vi "Na-DAS_7609.vi"() -> (0 "DAQ Error":errorcluster)   [LabVIEW 2015]
doc: "Use this plug-in with the Nathan 7609 data acquisition system"
uses:
  Globals/Meas_global.vi
  PWA/PWAtasksGLOBAL.vi
  Globals/Extra_Commands_Global.vi
  Globals/Dynamic_call_global.ph.vi
  Globals/Trav_pos_global.vi
panel:
  in  "Input voltage range (V)":u8(ring)=1 items=["-5... +5 V", "-10... +10 V"]
  out "Config read-back ok":bool
  out "Overruns":u32
  # "PN 25/11/2014, 19/12/2014, 15/02/2015 (channels in any order), 17/08/2015 (stop ack mod)"
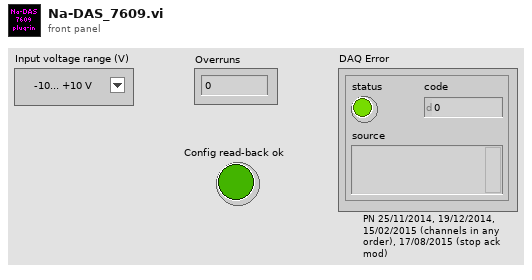
[diagram p1: front panel]
types:
  T1 = typedef "LDA_Setup.ctl" = cluster{"dimensions":enum16{"1D", "2D"}, "Analogue Freq Multiplier":dbl}
  T2 = typedef "Ch_and_Spans.ctl" = cluster{"high limit (10V)":sgl, "low limit (-10V)":sgl, "Ch No":i16, "Var name":string, "Use Latest Calib":bool}
  T3 = typedef "Traverse_cluster.ctl" = cluster{"Start X":sgl, "Start Y":sgl, "Start Z":sgl, "End X":sgl, "End Y":sgl, "End Z":sgl, "No. of pts.":i32, "Spacing":T4, "Filename":path, "Tunnel Speed":dbl, "Averaging time (min)":dbl, "Extra Commands":string, "Carrier_1 Q (l/min)":dbl, "Carrier_2 Q (l/min)":dbl, "Trace Gas Concentration (%)":dbl, "Specific Arguments":string, "Comments":string, "Row No":i32, "Row Type Selector":T5, "Completion time":string, "Row Duration (mins)":dbl, "No. of Valid pts.":i32, "Meas Setup File":string}
  T4 = typedef "Spacing.ctl" = enum16{"Linear", "Log", "Gauss", "Specified", "N/A"}
  T5 = typedef "Multi_run_mode.ctl" = enum16{"Move Traverse Only", "Set Tunnel Speed Only", "Set Source Only", "Set Measurement Conditions", "Single Measurement", "Vertical Profile", "Lateral Profile", "Longitudinal Profile", "Explore Volume", "Multi-Axis Profile", "Auto Calibrate", "Meas Fast FID Bkgnd", "Check Beam Power", "Scanning Valve Measurement", "Run VI Named:", "Set ADAM Ch", "Wait (minutes)", "Send Message", "Synchronize With:", "Fall Back to this Row", "Turn Off Row Repeating", "Blank Row", "Traverse 3D Volume"}
  T6 = typedef "Trigger_Mode.ctl" = enum16{"Free Running", "Start on Trigger", "Trigger Every Block", "Trigger Every Sample"}
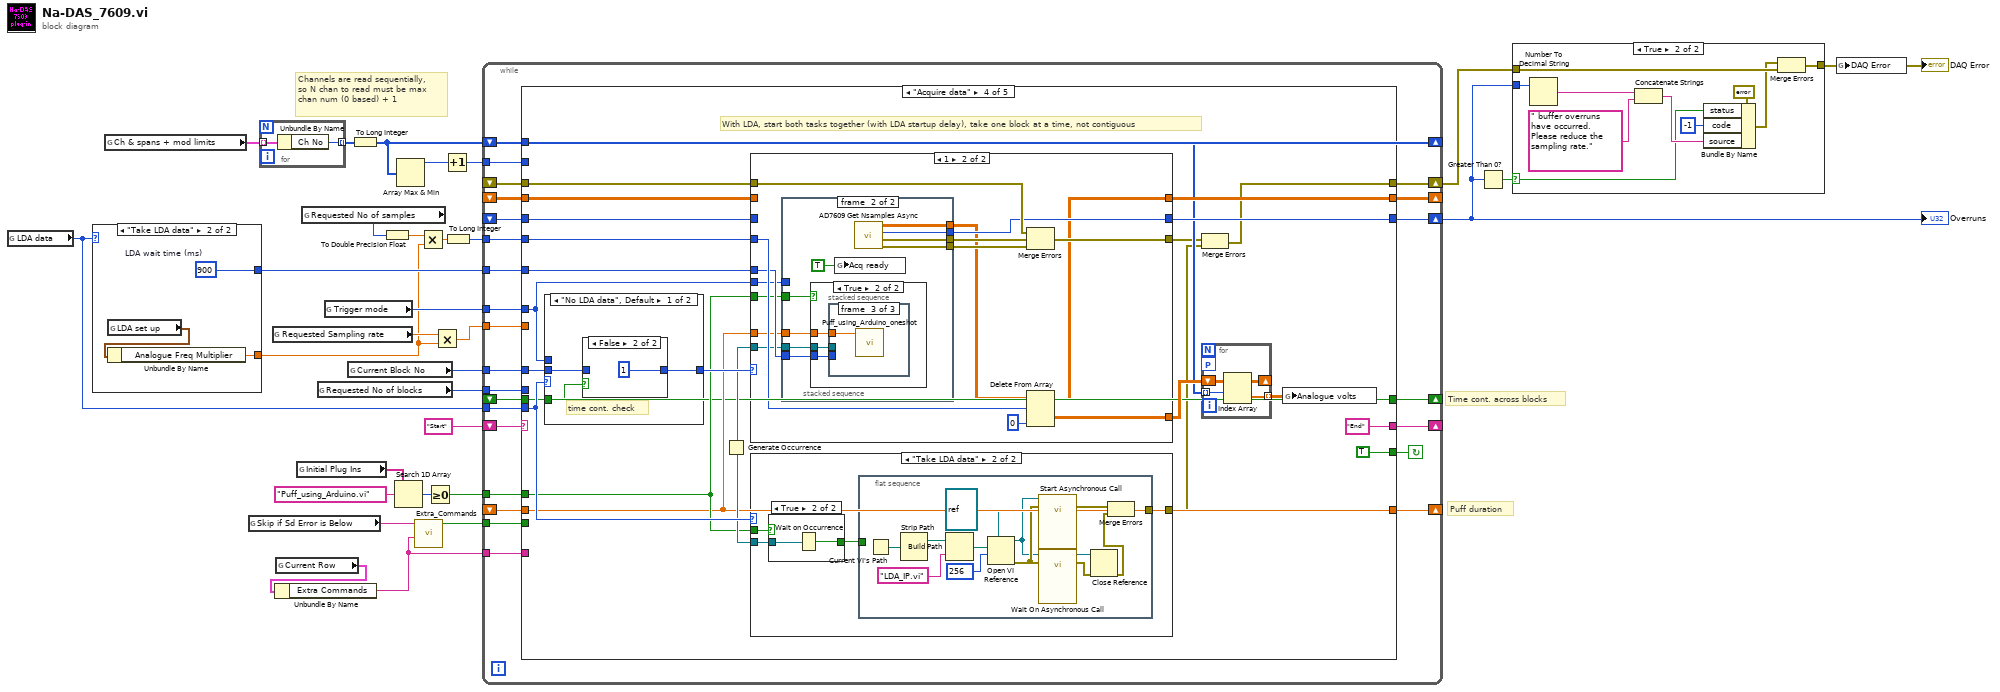
[diagram p0: block diagram]
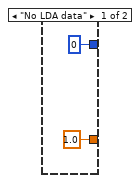
[diagram p3: hidden frame]
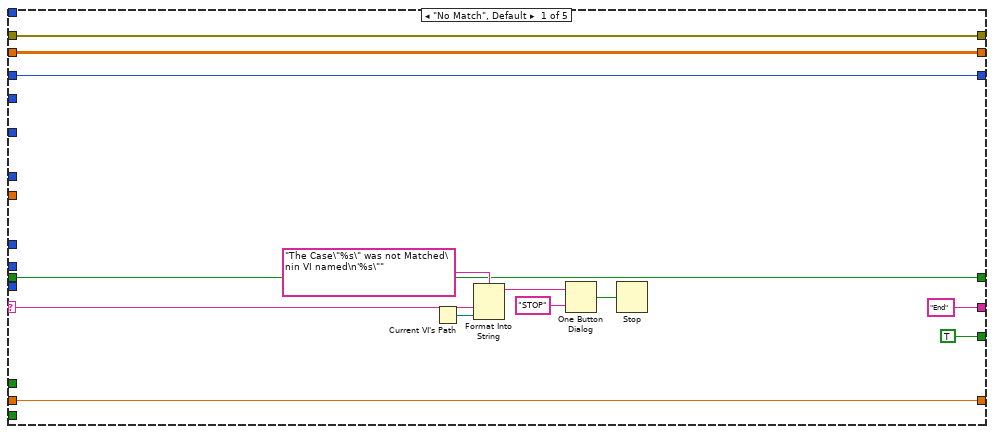
[diagram p4: hidden frame]
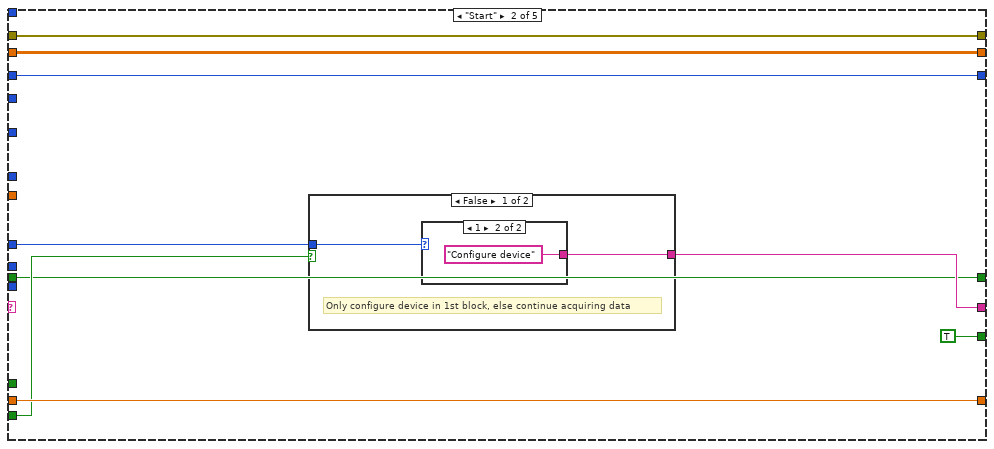
[diagram p5: hidden frame]
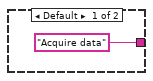
[diagram p6: hidden frame]
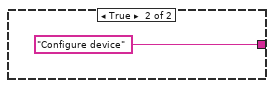
[diagram p7: hidden frame]
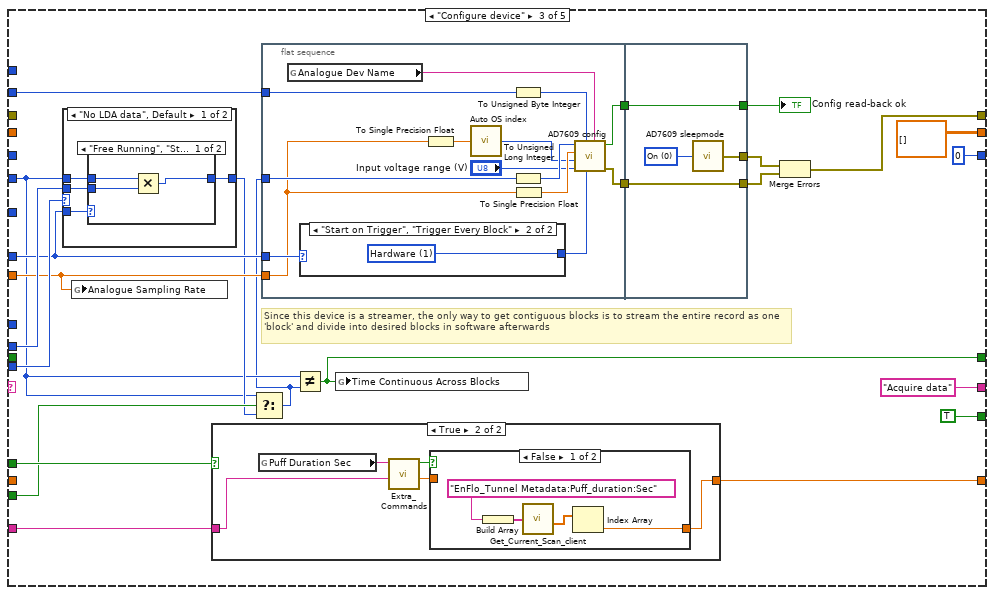
[diagram p8: hidden frame]
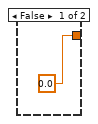
[diagram p9: hidden frame]
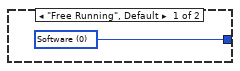
[diagram p13: hidden frame]
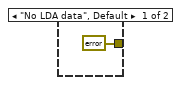
[diagram p14: hidden frame]
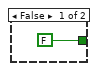
[diagram p15: hidden frame]
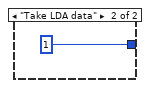
[diagram p17: hidden frame]
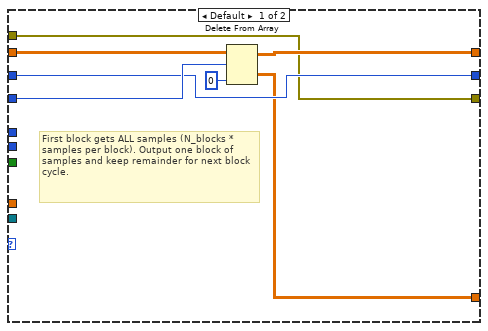
[diagram p18: hidden frame]
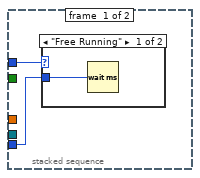
[diagram p19: hidden frame]
diagram:
  # "Time cont. across blocks"
  # "Puff duration"
  # "Channels are read sequentially, so N chan to read must be max chan num (0 based) + 1"
  n1 = global read "Meas_global.vi" "LDA data"() -> (w25:enum16{"No LDA data", "Take LDA data"})
  n2 = case shown="\"Take LDA data\"" w25 {
    tunnel: [1.0 ("Analogue Freq Multiplier") w34] -> w16
    tunnel: [u32 0 ("LDA wait time (ms)") w33] -> w20
    frame "No LDA data" {
    }
    frame "Take LDA data" {
      w33 = u32 900  # LDA wait time (ms)
      n3 = global read "Meas_global.vi" "LDA set up"() -> (w35:T1)
      n4 = Unbundle By Name(w35) -> ("Analogue Freq Multiplier"=w34:dbl)
    }
  }
  n5 = global read "Meas_global.vi" "Ch & spans + mod limits"() -> (w11:T2[])
  n6 = global read "Extra_Commands_Global.vi" "Skip if Sd Error is Below"() -> (w5:string)
  n7 = for {
    tunnel: w11 -> [w37] mode=indexing
    tunnel: [w36] -> w10 mode=indexing
    n8 = Unbundle By Name(w37) -> ("Ch No"=w36:i16)
  }
  n9 = global read "Meas_global.vi" "Requested Sampling rate"() -> (w26:dbl)
  n10 = global read "Trav_pos_global.vi" "Current Row"() -> (w6:T3)
  n11 = Unbundle By Name(w6) -> ("Extra Commands"=w4:string)
  n12 = global read "Dynamic_call_global.ph.vi" "Initial Plug Ins"() -> (w22:string[])
  n13 = global read "Meas_global.vi" "Requested No of samples"() -> (w17:i32)
  n14 = global read "Meas_global.vi" "Requested No of blocks"() -> (w13:i32)
  n15 = global read "Meas_global.vi" "Trigger mode"() -> (w29:T6)
  n16 = global read "Meas_global.vi" "Current Block No"() -> (w28:i32)
  n17 = To Long Integer(number=w10) -> (32bit integer=w9:i32[])
  n18 = To Double Precision Float(number=w17) -> (double precision float=w15:dbl)
  n19 = Search 1D Array(1D array=w22, element="Puff_using_Arduino.vi") -> (index of element=w24:i32)  [unwired: 1 in]
  n20 = Array Max & Min(array=w9) -> (max value=w8:i32)  [unwired: 3 out]
  n21 = call "Extra_Commands.vi"("String to Search"=w4, "Command"=w5) -> ("Command Found"=w3:bool)  [unwired: 2 in, 3 out]
  n22 = Multiply(x=w15, y=w16) -> (x*y=w14:dbl)
  n23 = Greater Or Equal To 0?(x=w24) -> (x >= 0?=w21:bool)
  n24 = Multiply(x=w26, y=w16) -> (x*y=w27:dbl)
  n25 = Increment(x=w8) -> (x+1=w7:i32)
  n26 = To Long Integer(number=w14) -> (32bit integer=w12:i32)
  n27 = while {
    shift-left: "Start" -> [w62]
    shift-right: [w48] -> _
    tunnel: w27 -> [w61]
    tunnel: w12 -> [w60]
    tunnel: w28 -> [w59]
    tunnel: w29 -> [w57]
    tunnel: w25 -> [w56]
    tunnel: w13 -> [w55]
    shift-right: [w53] -> w19
    shift-left: _ -> [w54]
    shift-right: [w52] -> _
    shift-left: _ -> [w51]
    shift-right: [w50] -> w1
    shift-left: _ -> [w49]
    tunnel: w20 -> [w47]
    tunnel: w21 -> [w46]
    shift-right: [w45] -> _
    shift-left: _ -> [w44]
    shift-right: [w43] -> _
    shift-left: w9 -> [w43]
    tunnel: w7 -> [w42]
    tunnel: w4 -> [w41]
    tunnel: w3 -> [w40]
    shift-right: [w39] -> _
    shift-left: _ -> [w38]
    stop <- w58 continue-if-true
    n28 = case shown="\"Acquire data\"" w62 {
      selector: w62 -> [w68 _ _ _ _]
      tunnel: ["End" w81 "Acquire data" ("f") "End" "End" ("f")] -> w48
      tunnel: w61 -> [_ _ w100 _ _]
      tunnel: w60 -> [_ _ w92 w170 _]
      tunnel: w59 -> [_ w82 _ w166 w253]
      tunnel: [TRUE TRUE TRUE TRUE FALSE] -> w58
      tunnel: w57 -> [_ _ w99 w160 _]
      tunnel: w56 -> [_ _ w110 w164 _]
      tunnel: w55 -> [_ _ w109 _ w254]
      tunnel: w54 -> [w67 w83 _ w173 w251]
      tunnel: [w67 w83 w111 w153 w250] -> w53
      tunnel: [w66 w80 dbl[][] [] ("Channel volts") w168 w249] -> w52
      tunnel: w51 -> [w66 w80 _ w169 w249]
      tunnel: [w65 w79 u32 0 ("Overruns") w172 w248] -> w50
      tunnel: w49 -> [w65 w79 _ w171 w248]
      tunnel: w47 -> [_ _ _ w165 _]
      tunnel: w46 -> [_ _ w98 w162 _]
      tunnel: [w64 w78 w97 w161 w247] -> w45
      tunnel: w44 -> [w64 w78 _ w161 w247]
      tunnel: w43 -> [_ _ _ w158 _]
      tunnel: w42 -> [_ _ w96 _ _]
      tunnel: w41 -> [_ _ w95 _ _]
      tunnel: w40 -> [_ w77 w94 _ _]
      tunnel: [w63 w76 w90 w156 w246] -> w39
      tunnel: w38 -> [w63 w76 _ w156 w246]
      frame "No Match", Default {
        n29 = Current VI's Path() -> (path=w71:path)
        n30 = Format Into String(format string="The Case\"%s\" was not Matched\nin VI named\n'%s\"" ("Format String"), w68, w71) -> (resulting string=w74:string)  [unwired: 2 in, 1 out]
        n31 = One Button Dialog(message=w74, button name ("OK")="STOP") -> (true=w72:bool)
        n32 = Stop(stop? (T)=w72) -> ()
      }
      frame "Start" {
        n33 = case shown="False" w77 {
          tunnel: w82 -> [w86 _]
          tunnel: [w85 "Configure device" ("f")] -> w81
          frame False {
            # "Only configure device in 1st block, else continue acquiring data"
            n34 = case shown="1" w86 {
              tunnel: ["Acquire data" ("f") "Configure device" ("f")] -> w85
              frame Default {
              }
              frame 1 {
              }
            }
          }
          frame True {
          }
        }
      }
      frame "Configure device" {
        # "Since this device is a streamer, the only way to get contiguous blocks is to stream the entire record as one 'block' and divide into desired blocks in software afterwards"
        n35 = case shown="\"No LDA data\", Default" w110 {
          tunnel: [w125 w132] -> w93
          tunnel: w92 -> [w127 w132]
          tunnel: w109 -> [w126 _]
          tunnel: w99 -> [w124 _]
          frame "No LDA data", Default {
            n36 = case shown="\"Free Running\", \"Start on Trigger\"" w124 {
              tunnel: w127 -> [w130 w131]
              tunnel: w126 -> [w129 _]
              tunnel: [w128 w131] -> w125
              frame "Free Running", "Start on Trigger" {
                n37 = Multiply(x=w130, y=w129) -> (x*y=w128:i32)
              }
              frame "Trigger Every Block", Default {
              }
            }
          }
          frame "Take LDA data" {
          }
        }
        n38 = global write "Meas_global.vi" "Analogue Sampling Rate"(w100) -> ()
        n39 = case shown="True" w98 {
          tunnel: [0.0 w118] -> w97
          tunnel: w95 -> [_ w114]
          frame False {
          }
          frame True {
            n40 = global read "Extra_Commands_Global.vi" "Puff Duration Sec"() -> (w117:string)
            n41 = call "Extra_Commands.vi"("String to Search"=w114, "Command"=w117) -> ("Numeric Value"=w115:dbl, "Command Found"=w116:bool)  [unwired: 2 in, 2 out]
            n42 = case shown="False" w116 {
              tunnel: [w119 w123] -> w118
              tunnel: w115 -> [_ w123]
              frame False {
                n43 = Build Array("EnFlo_Tunnel Metadata:Puff_duration:Sec") -> (w121:string[])
                n44 = call "Get_Current_Scan_client.vi"("ADAM Ch Names"=w121) -> ("Numerical Values"=w122:dbl[])  [unwired: 1 in, 2 out]
                n45 = Index Array(array=w122) -> (element=w119:dbl)  [unwired: 1 in]
              }
              frame True {
              }
            }
          }
        }
        n46 = Select(t=w92, s=w94, f=w93) -> (s? t:f=w91:i32)
        n47 = flat-sequence {
          tunnel: w91 -> [w146]
          tunnel: w100 -> [w136]
          tunnel: w99 -> [w145]
          tunnel: [w139] -> w108
          tunnel: [w138] -> w107
          tunnel: w96 -> [w133]
          tunnel: [w151] -> w104
          tunnel: w108 -> [w151]
          tunnel: [w150] -> w106
          tunnel: w107 -> [w150]
          tunnel: [w149] -> w105
          frame #0 {
            n48 = global read "PWAtasksGLOBAL.vi" "Analogue Dev Name"() -> (w144:string)
            n49 = case shown="\"Start on Trigger\", \"Trigger Every Block\"" w145 {
              tunnel: [w147 w148] -> w141
              frame "Free Running", Default {
                w147 = u8 0 items=["Software", "Hardware"] ("Triggering mode")
              }
              frame "Start on Trigger", "Trigger Every Block" {
                w148 = u8 1 items=["Software", "Hardware"] ("Triggering mode")
              }
            }
            n50 = To Single Precision Float(number=w136) -> (single precision float=w134:sgl)
            n51 = call "Auto OS index.vi"("Sampling rate"=w134) -> ("OS index"=w135:u8)
            n52 = To Unsigned Byte Integer(number=w133) -> (unsigned 8bit integer=w140:u8)
            n53 = To Unsigned Long Integer(number=w146) -> (unsigned 32bit integer=w143:u32)
            n54 = To Single Precision Float(number=w136) -> (single precision float=w142:sgl)
            n55 = call "AD7609 config.vi"("Device serial port"=w144, "Triggering mode"=w141, "N channels to read"=w140, "Input voltage range (V)"="Input voltage range (V)", "Oversampling ratio"=w135, "Sampling rate (Hz)"=w142, "Number of samples"=w143) -> ("Config error out"=w138:errorcluster, "Config read-back ok"=w139:bool)  [unwired: 3 in]
          }
          frame #1 {
            w152 = u8 0 items=["On", "Standby", "Shutdown"] ("Sleep state")
            n56 = call "AD7609 sleepmode.vi"("Sleep state"=w152) -> ("Sleep error out"=w149:errorcluster)
          }
        }
        n57 = Not Equal?(x=w92, y=w91) -> (x != y?=w90:bool)
        n58 = global write "Meas_global.vi" "Time Continuous Across Blocks"(w90) -> ()
        n59 = Merge Errors(w105, w106) -> (w111:errorcluster)
        "Config read-back ok" <- w104
      }
      frame "Acquire data" {
        # "With LDA, start both tasks together (with LDA startup delay), take one block at a time, not contiguous"
        n60 = case shown="\"No LDA data\", Default" w164 {
          tunnel: w166 -> [w201 _]
          tunnel: w160 -> [_ _]
          tunnel: [w202 1 ("Current Block No")] -> w167
          tunnel: w156 -> [w200 _]
          frame "No LDA data", Default {
            # "time cont. check"
            n61 = case shown="False" w200 {
              tunnel: [w203 1 ("Current Block No")] -> w202
              tunnel: w201 -> [w203 _]
              frame True {
              }
              frame False {
              }
            }
          }
          frame "Take LDA data" {
          }
        }
        n62 = Generate Occurrence() -> (w163:refnum<k4>)
        n63 = case shown="1" w167 {
          tunnel: w173 -> [w207 w225]
          tunnel: [w207 w224] -> w155
          tunnel: [w208 w223] -> w172
          tunnel: [w210 w220] -> w168
          tunnel: w170 -> [w209 w221]
          tunnel: w169 -> [w211 _]
          tunnel: w171 -> [w208 _]
          tunnel: [w206 w218] -> w159
          tunnel: w165 -> [_ w217]
          tunnel: w163 -> [_ w216]
          tunnel: w162 -> [_ w215]
          tunnel: w161 -> [_ w214]
          tunnel: w160 -> [_ w213]
          frame Default {
            # "First block gets ALL samples (N_blocks * samples per block). Output one block of samples and keep remainder for next block cycle."
            n64 = Delete From Array(array=w211, length=w209, index (col)=0 ("disabled index (col)")) -> (deleted portion=w206:dbl[][], array with subset deleted=w210:dbl[][])  [unwired: 1 in]
          }
          frame 1 {
            n65 = stacked-sequence {
              tunnel: [_ w238] -> w223
              tunnel: [_ w237] -> w222
              tunnel: [_ w236] -> w227
              tunnel: [_ w235] -> w226
              tunnel: w216 -> [_ w234]
              tunnel: w217 -> [w229 w233]
              tunnel: w215 -> [_ w232]
              tunnel: w214 -> [_ w231]
              tunnel: w213 -> [w228 _]
              frame #0 {
                n66 = case shown="\"Free Running\"" w228 {
                  tunnel: w229 -> [w230 _]
                  frame "Free Running" {
                    n67 = Wait (ms)(milliseconds to wait=w230) -> ()  [unwired: 1 out]
                  }
                  frame Default {
                  }
                }
              }
              frame #1 {
                n68 = case shown="True" w232 {
                  tunnel: w234 -> [_ w242]
                  tunnel: w231 -> [_ w241]
                  tunnel: w233 -> [_ w240]
                  frame False {
                  }
                  frame True {
                    n69 = stacked-sequence {
                      tunnel: w242 -> [w243 _ _]
                      tunnel: w241 -> [_ _ w245]
                      tunnel: w240 -> [_ w244 _]
                      frame #0 {
                        n70 = Set Occurrence(w243) -> ()
                      }
                      frame #1 {
                        n71 = Wait (ms)(milliseconds to wait=w244) -> ()  [unwired: 1 out]
                      }
                      frame #2 {
                        n72 = call "Puff_using_Arduino_oneshot.vi"("Puff_duration:Sec"=w245) -> ()  [unwired: 7 in]
                      }
                    }
                  }
                }
                n73 = global write "Meas_global.vi" "Acq ready"(TRUE ("Acq ready")) -> ()
                n74 = call "AD7609 Get Nsamples Async.vi"() -> ("Channel volts"=w237:dbl[][], "Overruns"=w238:u32, "Async error"=w235:errorcluster, "Overrun error out"=w236:errorcluster)  [unwired: 1 in]
              }
            }
            n75 = Merge Errors(w225, w226, w227) -> (w224:errorcluster)
            n76 = Delete From Array(array=w222, length=w221, index (col)=0 ("disabled index (col)")) -> (deleted portion=w218:dbl[][], array with subset deleted=w220:dbl[][])  [unwired: 1 in]
          }
        }
        n77 = case shown="\"Take LDA data\"" w164 {
          tunnel: w162 -> [_ w183]
          tunnel: w163 -> [_ w181]
          tunnel: [errorcluster {"status"=FALSE, "code"=0, "source"=""} ("error IO") w180] -> w154
          frame "No LDA data", Default {
          }
          frame "Take LDA data" {
            n78 = case shown="True" w183 {
              tunnel: w181 -> [_ w186]
              tunnel: [FALSE ("timed out") w185] -> w182
              frame False {
              }
              frame True {
                n79 = Wait on Occurrence(2:w186) -> (0:w185:bool)  [unwired: 2 in]
              }
            }
            n80 = flat-sequence {
              tunnel: w182 -> [_]
              tunnel: [w187] -> w180
              frame #0 {
                n81 = Current VI's Path() -> (path=w197:path)
                n82 = Strip Path(path=w197) -> (stripped path=w196:path)  [unwired: 1 out]
                n83 = Build Path(base path=w196, name or relative path="LDA_IP.vi") -> (appended path=w198:path)
                n84 = Open VI Reference(type specifier VI Refnum (for type only)=refnum<vi> refnum, vi path=w198, options=256) -> (vi reference=w192:refnum<vi>, error out=w193:errorcluster)  [unwired: 3 in]
                n85 = call-by-ref "Start Asynchronous Call"(reference=w192, error in=w193) -> (error out=w189:errorcluster)  [unwired: 1 in, 2 out]
                n86 = call-by-ref "Wait On Asynchronous Call"(reference=w192, error in=w193) -> (reference out=w191:refnum<vi>, error out=w190:errorcluster)  [unwired: 1 in, 1 out]
                n87 = Close Reference(reference=w191, error in (no error)=w190) -> (error out=w188:errorcluster)
                n88 = Merge Errors(w189, w188) -> (w187:errorcluster)
              }
            }
          }
        }
        n89 = Merge Errors(w155, w154) -> (w153:errorcluster)
        n90 = for {
          shift-right: [w178] -> _
          shift-left: w159 -> [w178]
          tunnel: w158 -> [w176] mode=indexing
          tunnel: [w177] -> w157 mode=indexing
          workers-P: _ -> [_]
          n91 = Index Array(array=w178, index (row)=w176) -> (element=w177:dbl[])  [unwired: 1 in]
        }
        n92 = global write "Meas_global.vi" "Analogue volts"(w157) -> ()
      }
      frame "End" {
        n93 = Equal?(x=w253, y=w254) -> (x = y?=w252:bool)
        n94 = case shown="True" w252 {
          tunnel: w251 -> [w258 w260]
          tunnel: [w258 w259] -> w250
          frame False {
          }
          frame True {
            w262 = u8 1 items=["On", "Standby", "Shutdown"] ("Sleep state")
            n95 = call "AD7609 sleepmode.vi"("Sleep state"=w262) -> ("Sleep error out"=w261:errorcluster)
            n96 = Merge Errors(w260, w261) -> (w259:errorcluster)
          }
        }
        n97 = global write "Meas_global.vi" "Acq ready"(FALSE ("Acq ready")) -> ()
      }
    }
  }
  "Overruns" <- w1
  n98 = Greater Than 0?(x=w1) -> (x > 0?=w2:bool)
  n99 = case shown="True" w2 {
    selector: w2 -> [_ w265]
    tunnel: w19 -> [w263 w272]
    tunnel: [w263 w273] -> w18
    tunnel: w1 -> [_ w271]
    frame False {
    }
    frame True {
      n100 = Number To Decimal String(number=w271) -> (decimal integer string=w269:string)  [unwired: 1 in]
      n101 = Concatenate Strings(w269, " buffer overruns have occurred. Please reduce the sampling rate.") -> (w267:string)
      n102 = Bundle By Name(cluster=errorcluster {"status"=FALSE, "code"=0, "source"=""} ("error IO"), "status"=w265, "code"=-1, "source"=w267) -> (w264:errorcluster)
      n103 = Merge Errors(w264, w272) -> (w273:errorcluster)
    }
  }
  "DAQ Error" <- w18
  n104 = global write "Meas_global.vi" "DAQ Error"(w18) -> ()
